vi "Report.vi"(8 "error in (no error)":errorcluster {"code" format="Error %.0f"}, 10 "Full Documentation":T1, 11 "VIDoc Printer In":refnum<class "VIDoc Printer.lvclass">) -> (0 "error out":errorcluster {"code" format="Error %.0f"}, 3 "VIDoc Printer Out":refnum<class "VIDoc Printer.lvclass">)   [LabVIEW 2023, in "VIDoc Printer.lvlib" / "VIDoc Printer.lvclass"]
doc: "Takes in the Full Documentation cluster and runs the Printer on it."
uses:
  VIDoc Printer.lvclass
  VIDoc Printer.lvclass/VIDoc Printer.ctl
  Parsing/Project Documentation/Project Documentation.lvclass
  Parsing/Interface Documenation/Interface Documenation.lvclass
  Parsing/Class Documentation/Class Documentation.lvclass
  Parsing/Library Documentation/Library Documentation.lvclass
  Parsing/GUI Documentation/GUI Documentation.lvclass
  Parsing/TypeDefs/Full Documentation Info.ctl
  Parsing/VIDoc Parsing.lvlib
  Parsing/LLB Documentation/LLB Documentation.lvclass
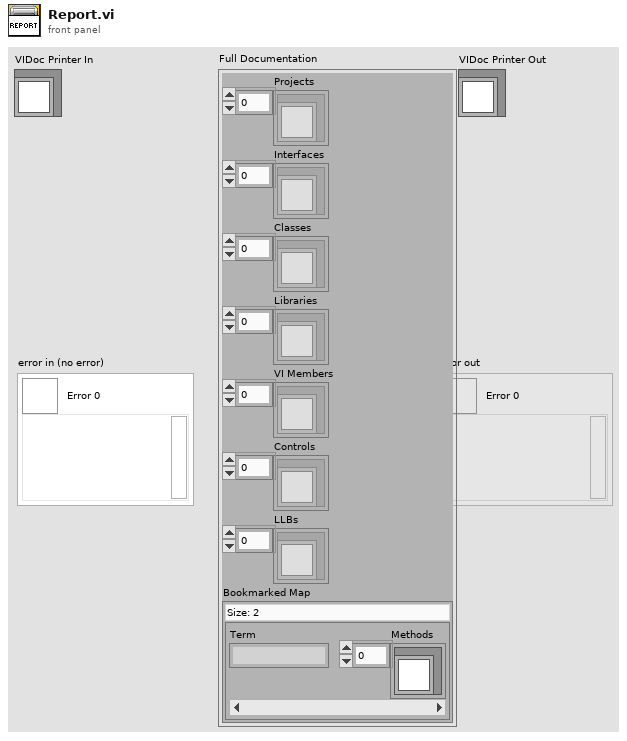
[diagram p1: front panel]
types:
  T1 = typedef "VIDoc Parsing.lvlib/Full Documentation Info.ctl" = cluster{"Projects":refnum<class "Project Documentation.lvclass">[], "Interfaces":refnum<class "Interface Documenation.lvclass">[], "Classes":refnum<class "Class Documentation.lvclass">[], "Libraries":refnum<class "Library Documentation.lvclass">[], "VI Members":refnum<class "GUI Documentation.lvclass">[], "Controls":refnum<class "GUI Documentation.lvclass">[], "LLBs":refnum<class "LLB Documentation.lvclass">[], "Bookmarked Map":map{string, refnum<class "GUI Documentation.lvclass">[]}}
  T2 = map{string, refnum<class "GUI Documentation.lvclass">[]}
  T3 = typedef "VIDoc Parsing.lvlib/Memory Size Cluster.ctl" = cluster{"Bookmarked":dbl, "Class":dbl, "Library":dbl, "VI":dbl, "Control":dbl}
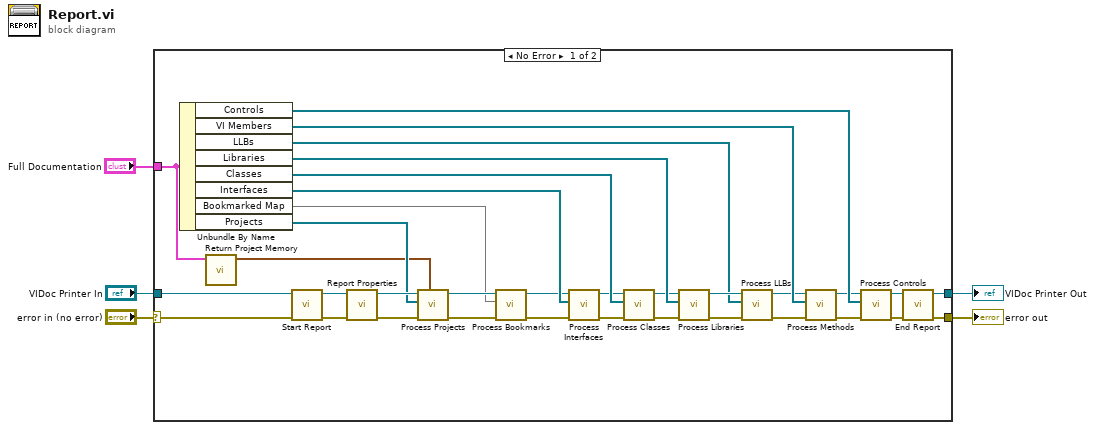
[diagram p0: block diagram]
diagram:
  n1 = case shown="No Error" "error in (no error)" {
    selector: "error in (no error)" -> [w35 w41]
    tunnel: [w33 w41] -> w4
    tunnel: [w32 w40] -> w2
    tunnel: "VIDoc Printer In" -> [w34 w40]
    tunnel: "Full Documentation" -> [w21 _]
    frame No Error {
      n2 = Unbundle By Name(w21) -> ("Controls"=w22:refnum<class "GUI Documentation.lvclass">[], "VI Members"=w23:refnum<class "GUI Documentation.lvclass">[], "LLBs"=w9:refnum<class "LLB Documentation.lvclass">[], "Libraries"=w24:refnum<class "Library Documentation.lvclass">[], "Classes"=w25:refnum<class "Class Documentation.lvclass">[], "Interfaces"=w26:refnum<class "Interface Documenation.lvclass">[], "Bookmarked Map"=w6:T2, "Projects"=w31:refnum<class "Project Documentation.lvclass">[])
      n3 = call "Return Project Memory.vi"("Full Documentation"=w21) -> ("Memory"=w20:T3)  [unwired: 10 in]
      n4 = call-dynamic "Start Report.vi"("error in (no error)"=w35, "VIDoc Printer In"=w34) -> ("error out"=w38:errorcluster, "VIDoc Printer Out"=w39:refnum<class "VIDoc Printer.lvclass">)  [unwired: 8 in]
      n5 = call-dynamic "Report Properties.vi"("error in (no error)"=w38, "VIDoc Printer In"=w39) -> ("error out"=w36:errorcluster, "VIDoc Printer Out"=w37:refnum<class "VIDoc Printer.lvclass">)  [unwired: 8 in]
      n6 = call-dynamic "Process Projects.vi"("Total Memory"=w20, "error in (no error)"=w36, "Projects"=w31, "VIDoc Printer In"=w37) -> ("error out"=w29:errorcluster, "VIDoc Printer Out"=w30:refnum<class "VIDoc Printer.lvclass">)  [unwired: 6 in]
      n7 = call-dynamic "Process Bookmarks.vi"("error in (no error)"=w29, "Bookmarked Map"=w6, "VIDoc Printer In"=w30) -> ("error out"=w8:errorcluster, "VIDoc Printer Out"=w7:refnum<class "VIDoc Printer.lvclass">)  [unwired: 7 in]
      n8 = call-dynamic "Process Interfaces.vi"("error in (no error)"=w8, "Interfaces"=w26, "VIDoc Printer In"=w7) -> ("error out"=w18:errorcluster, "VIDoc Printer Out"=w19:refnum<class "VIDoc Printer.lvclass">)  [unwired: 7 in]
      n9 = call-dynamic "Process Classes.vi"("error in (no error)"=w18, "Classes"=w25, "VIDoc Printer In"=w19) -> ("error out"=w16:errorcluster, "VIDoc Printer Out"=w17:refnum<class "VIDoc Printer.lvclass">)  [unwired: 7 in]
      n10 = call-dynamic "Process Libraries.vi"("error in (no error)"=w16, "Libraries"=w24, "VIDoc Printer In"=w17) -> ("error out"=w15:errorcluster, "VIDoc Printer Out"=w11:refnum<class "VIDoc Printer.lvclass">)  [unwired: 7 in]
      n11 = call-dynamic "Process LLBs.vi"("error in (no error)"=w15, "LLBs"=w9, "VIDoc Printer In"=w11) -> ("error out"=w12:errorcluster, "VIDoc Printer Out"=w10:refnum<class "VIDoc Printer.lvclass">)  [unwired: 7 in]
      n12 = call-dynamic "Process Methods.vi"("error in (no error)"=w12, "UIs"=w23, "VIDoc Printer In"=w10) -> ("error out"=w13:errorcluster, "VIDoc Printer Out"=w14:refnum<class "VIDoc Printer.lvclass">)  [unwired: 7 in]
      n13 = call-dynamic "Process Controls.vi"("error in (no error)"=w13, "Controls"=w22, "VIDoc Printer In"=w14) -> ("error out"=w27:errorcluster, "VIDoc Printer Out"=w28:refnum<class "VIDoc Printer.lvclass">)  [unwired: 7 in]
      n14 = call-dynamic "End Report.vi"("error in (no error)"=w27, "VIDoc Printer In"=w28) -> ("error out"=w33:errorcluster, "VIDoc Printer Out"=w32:refnum<class "VIDoc Printer.lvclass">)  [unwired: 8 in]
    }
    frame Error {
    }
  }
  "error out" <- w4
  "VIDoc Printer Out" <- w2
